vi "cycle_send_goal.vi"() -> ()   [LabVIEW 2014]
uses:
  <userlib>/ROS for LabVIEW Software/ROS/Code/Console/Servers/ServerSubs/TopicDef.ctl
  <userlib>/ROS for LabVIEW Software/ROS/Code/SubVIs/_ROSDirection.ctl
  ctl/Point.ctl
  ROS-for-LabVIEW-Software/MoreExample/ctl/pose.ctl
  ctl/RPY.ctl
panel:
  in  "set_vel":bool
  in  "pose":bool
  in  "cancel":bool
  in  "stop":bool
  in  "sent":bool
  out "error out":errorcluster
  out "Quaternion":cluster{"x":dbl, "y":dbl, "z":dbl, "w":dbl}
  out "what I sent msg out":string
  # "cannot connect one node in ONE vi in LabVIEW"
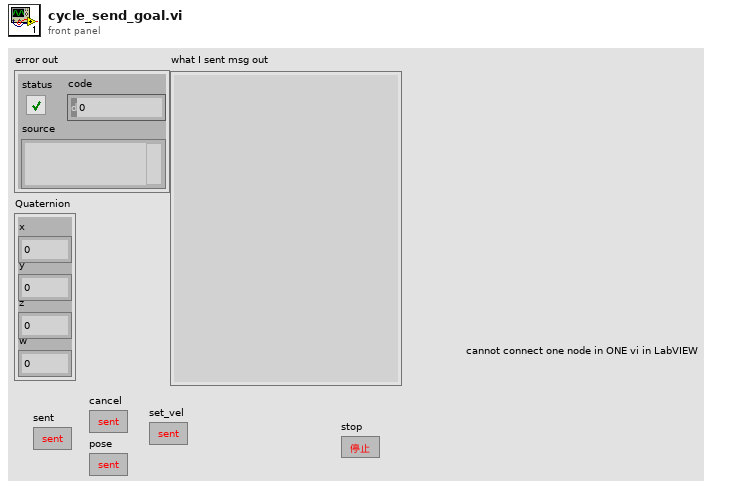
[diagram p1: front panel]
types:
  T1 = typedef "TopicDef.ctl" = cluster{"Topic":string, "Type":string, "Action":T2, "Update (ms)":u16, "queue size":u16}
  T2 = typedef "_ROSDirection.ctl" = enum16{"Node", "Publisher", "Subscriber", "ServiceClient", "ServiceProvider"}
  T3 = typedef "_ROSControl.ctl" = cluster{"topic port":u16, "Node":string, "topic":string, "type":string, "node port":u16, "error ":errorcluster, "Direction":T2, "Update (ms)":u16, "FIFO size":u16}
  T4 = typedef "RPY.ctl" = cluster{"Roll (y)":dbl, "Pitch (x)":dbl, "Yaw (z)":dbl}
  T5 = typedef "pose.ctl" = cluster{"Point":cluster{"x":dbl, "y":dbl, "z":dbl}, "Quaternion":cluster{"x":dbl, "y":dbl, "z":dbl, "w":dbl}}
  T6 = typedef "Point.ctl" = cluster{"x":dbl, "y":dbl, "z":dbl}
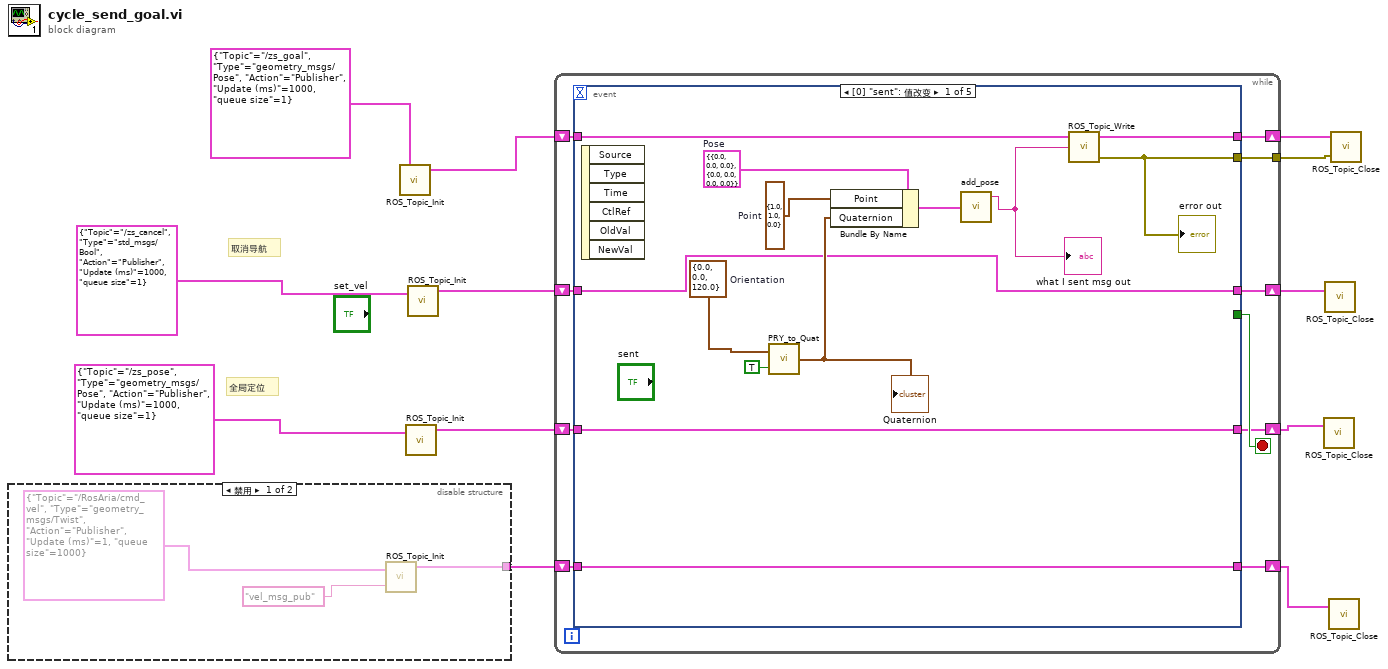
[diagram p0: block diagram]
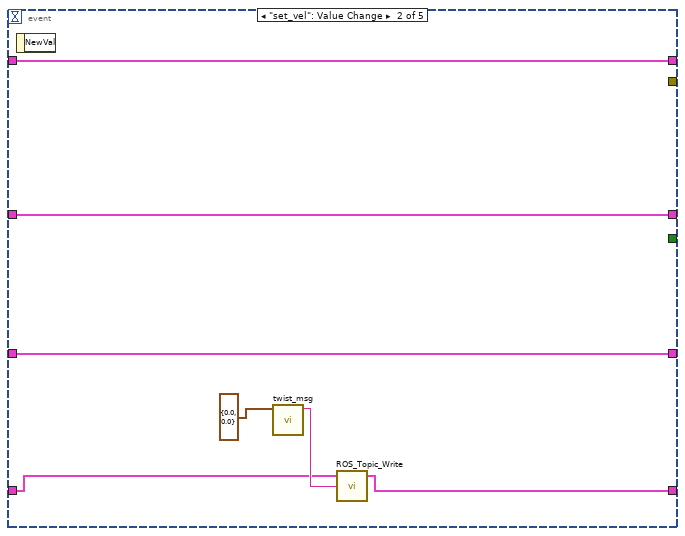
[diagram p3: hidden frame]
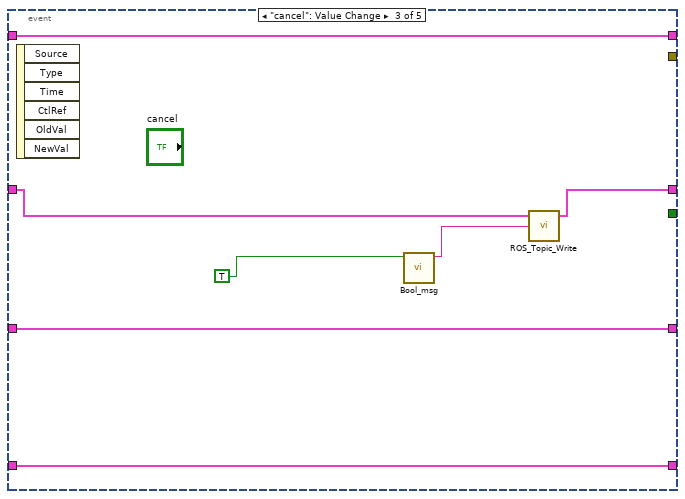
[diagram p4: hidden frame]
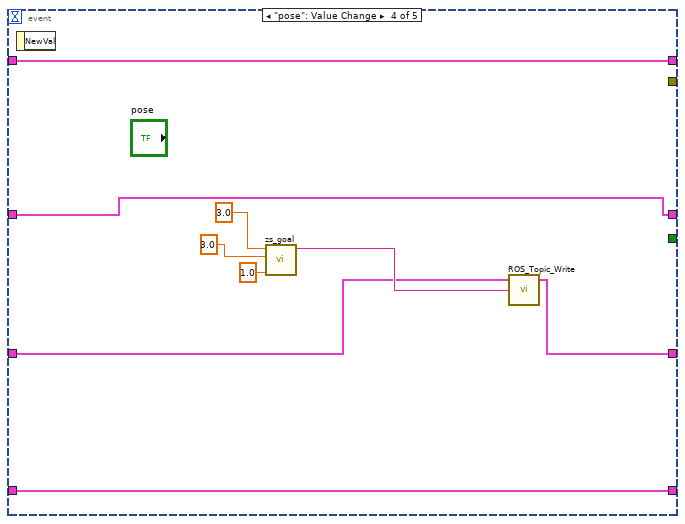
[diagram p5: hidden frame]
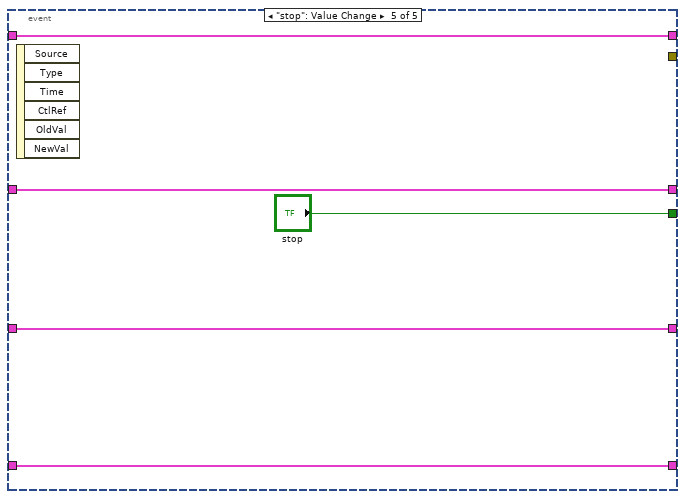
[diagram p6: hidden frame]
diagram:
  # "全局定位"
  # "取消导航"
  n1 = disable-structure shown="禁用" {
    disable-tunnel: [w15 _] -> w4
    frame Disabled {
      n2 = call <userlib>:"ROS_Topic_Init.vi"("Definitions"=T1 {"Topic"="/RosAria/cmd_vel", "Type"="geometry_msgs/Twist", "Action"=enum."Publisher", "Update (ms)"=1, "queue size"=1000}, "node"="vel_msg_pub") -> ("ROS out"=w15:T3)  [unwired: 1 in, 1 out]
    }
    frame Enabled {
    }
  }
  n3 = call <userlib>:"ROS_Topic_Init.vi"("Definitions"=T1 {"Topic"="/zs_goal", "Type"="geometry_msgs/Pose", "Action"=enum."Publisher", "Update (ms)"=1000, "queue size"=1}) -> ("ROS out"=w9:T3)  [unwired: 2 in, 1 out]
  n4 = call <userlib>:"ROS_Topic_Init.vi"("Definitions"=T1 {"Topic"="/zs_pose", "Type"="geometry_msgs/Pose", "Action"=enum."Publisher", "Update (ms)"=1000, "queue size"=1}) -> ("ROS out"=w7:T3)  [unwired: 2 in, 1 out]
  n5 = call <userlib>:"ROS_Topic_Init.vi"("Definitions"=T1 {"Topic"="/zs_cancel", "Type"="std_msgs/Bool", "Action"=enum."Publisher", "Update (ms)"=1000, "queue size"=1}) -> ("ROS out"=w8:T3)  [unwired: 2 in, 1 out]
  n6 = while {
    tunnel: [w25] -> w12
    shift-right: [w24] -> w11
    shift-left: w9 -> [w23]
    shift-right: [w20] -> w5
    shift-left: w8 -> [w21]
    shift-right: [w18] -> w6
    shift-left: w7 -> [w19]
    shift-right: [w16] -> w3
    shift-left: w4 -> [w17]
    stop <- w22 stop-if-true
    n7 = event shown="[0] \"sent\": 值改变" {
      selector: _ -> [_ _ _ _ _]
      dyn-events: _ -> [_ _ _ _ _]
      timeout: _ -> [_ _ _ _ _]
      tunnel: [w38 _ _ _ _] -> w25
      tunnel: [w37 w39 w48 w55 w65] -> w24
      tunnel: w23 -> [w36 w39 w48 w55 w65]
      tunnel: [_ _ _ _ "stop"] -> w22
      tunnel: w21 -> [w28 w40 w50 w54 w64]
      tunnel: [w28 w40 w49 w54 w64] -> w20
      tunnel: w19 -> [w27 w41 w47 w57 w63]
      tunnel: [w27 w41 w47 w56 w63] -> w18
      tunnel: w17 -> [w26 w43 w46 w53 w62]
      tunnel: [w26 w42 w46 w53 w62] -> w16
      event "sent": Value Change {
        w34 = T4 {"Roll (y)"=0.0, "Pitch (x)"=0.0, "Yaw (z)"=120.0}  # Orientation
        w33 = T5 {"Point"={"x"=0.0, "y"=0.0, "z"=0.0}, "Quaternion"={"x"=0.0, "y"=0.0, "z"=0.0, "w"=0.0}}  # Pose
        w32 = T6 {"x"=1.0, "y"=1.0, "z"=0.0}  # Point
        n8 = event-data() -> ()  [unwired: 1 in, 6 out]
        n9 = call <userlib>:"PRY_to_Quat.vi"("From Degrees? (T)"=TRUE, "Orientation"=w34) -> ("Quaternion"=w31:cluster{"x":dbl, "y":dbl, "z":dbl, "w":dbl})
        "Quaternion" <- w31
        n10 = Bundle By Name(cluster=w33, "Point"=w32, "Quaternion"=w31) -> (w29:T5)
        n11 = call <userlib>:"add_pose.vi"("Pose"=w29) -> ("msg out"=w30:string)  [unwired: 4 in]
        "what I sent msg out" <- w30
        n12 = call <userlib>:"ROS_Topic_Write.vi"("Msg in"=w30, "ROS in"=w36) -> ("error out"=w38:errorcluster, "ROS out"=w37:T3)  [unwired: 2 in]
        "error out" <- w38
      }
      event "set_vel": Value Change {
        n13 = event-data() -> ()  [unwired: 1 in, 1 out]
        n14 = call "twist_msg.vi"("vel_cal"=cluster{"rot_z":dbl, "lin_x":dbl} {"rot_z"=0.0, "lin_x"=0.0} ("值")) -> ("msg out"=w44:string)  [unwired: 10 in]
        n15 = call <userlib>:"ROS_Topic_Write.vi"("Msg in"=w44, "ROS in"=w43) -> ("ROS out"=w42:T3)  [unwired: 2 in, 1 out]
      }
      event "cancel": Value Change {
        n16 = event-data() -> ()  [unwired: 1 in, 6 out]
        n17 = call "Bool_msg.vi"("Boolean"=TRUE) -> ("msg out"=w52:string)  [unwired: 10 in]
        n18 = call <userlib>:"ROS_Topic_Write.vi"("Msg in"=w52, "ROS in"=w50) -> ("ROS out"=w49:T3)  [unwired: 2 in, 1 out]
      }
      event "pose": Value Change {
        n19 = event-data() -> ()  [unwired: 1 in, 1 out]
        n20 = call "zs_goal.vi"("Yaw (z)"=1.0, "Point.y"=3.0, "Point.x"=3.0) -> ("msg out"=w61:string)  [unwired: 8 in]
        n21 = call <userlib>:"ROS_Topic_Write.vi"("Msg in"=w61, "ROS in"=w57) -> ("ROS out"=w56:T3)  [unwired: 2 in, 1 out]
      }
      event "stop": Value Change {
        n22 = event-data() -> ()  [unwired: 1 in, 6 out]
      }
    }
  }
  n23 = call <userlib>:"ROS_Topic_Close.vi"("ROS in"=w6) -> ()  [unwired: 3 in, 1 out]
  n24 = call <userlib>:"ROS_Topic_Close.vi"("ROS in"=w5) -> ()  [unwired: 3 in, 1 out]
  n25 = call <userlib>:"ROS_Topic_Close.vi"("ROS in"=w3) -> ()  [unwired: 3 in, 1 out]
  n26 = call <userlib>:"ROS_Topic_Close.vi"("error in"=w12, "ROS in"=w11) -> ()  [unwired: 2 in, 1 out]
